vi "Update Normalized Axes Logic.vi"(8 "axis":i32, 11 "axis in":dbl[](array[numeric])) -> (3 "axis out":dbl[](array[numeric]))   [LabVIEW 2012]
doc: "This VI contains specific logic to update an individual axis' minimum and maximum range.\nRuffin"
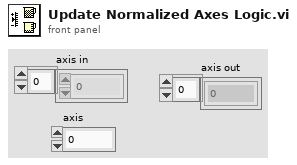
[diagram p1: front panel]
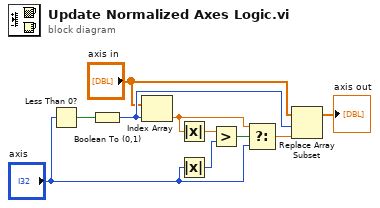
[diagram p0: block diagram]
diagram:
  n1 = Less Than 0?(x="axis") -> (x < 0?=w10:bool)
  n2 = Boolean To (0,1)(Boolean=w10) -> (0, 1=w5:i16)
  n3 = Index Array(array="axis in", index=w5) -> (element=w6:dbl)
  n4 = Absolute Value(x=w6) -> (abs(x)=w8:dbl)
  n5 = Absolute Value(x="axis") -> (abs(x)=w7:i32)
  n6 = Greater?(x=w8, y=w7) -> (0:w9:bool)
  n7 = Select(t=w6, s=w9, f="axis") -> (s? t:f=w4:dbl)
  n8 = Replace Array Subset(array="axis in", new element=w4, index=w5) -> (→"axis out":dbl[])
